vi "Add Stream.vi"(6 "Pixel Fornat || Options":u32, 8 "error in (no error)":errorcluster, 9 "Desired Stream Parameters":T1, 10 "Device ID":string, 11 "CameraManager":refnum<data-value>) -> (0 "error out":errorcluster, 2 "Stream":refnum<data-value>, 3 "CameraManager (duplicate)":refnum<data-value>)   [LabVIEW 2020, in "g_ar_toolkit.capture.lvlib" / "CameraManager.lvclass"]
uses:
  CameraManager.lvclass
  Stream Parameters.ctl
  CameraStream/CameraStream.lvclass
  CameraManager.lvclass/CameraManager.ctl
  bin/g_ar_toolkit.1.32.dll
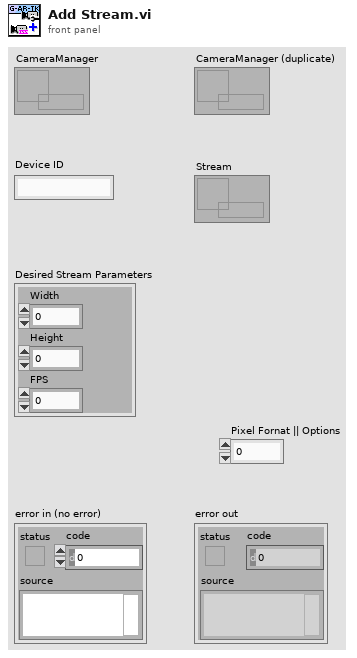
[diagram p1: front panel]
types:
  T1 = typedef "g_ar_toolkit.capture.lvlib/CameraManager.lvclass/Stream Parameters.ctl" = cluster{"Width":u16, "Height":u16, "FPS":u8}
  T2 = cluster{"Width":u32, "Height":u32, "FPS":u32, u32}
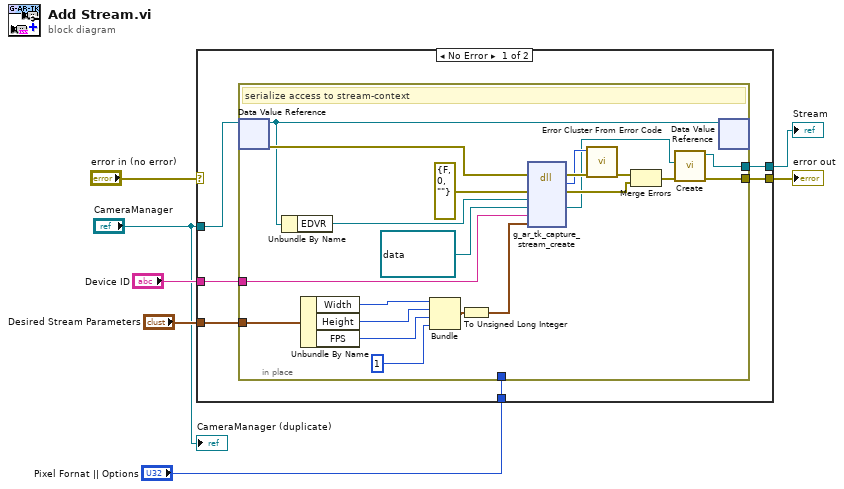
[diagram p0: block diagram]
diagram:
  n1 = case shown="No Error" "error in (no error)" {
    selector: "error in (no error)" -> [_ w35]
    tunnel: "CameraManager" -> [w13 _]
    tunnel: "Device ID" -> [w12 _]
    tunnel: "Desired Stream Parameters" -> [w11 _]
    tunnel: [w10 _] -> w4
    tunnel: [w9 w35] -> w3
    tunnel: "Pixel Fornat || Options" -> [w8 _]
    frame No Error {
      n2 = in-place {
        in-place-border: w12 -> [w30]
        in-place-border: w11 -> [w16]
        in-place-border: [w19] -> w10
        in-place-border: [w18] -> w9
        in-place-border: w8 -> [_]
        # "serialize access to stream-context"
        n3 = in-place-dvr #1(w13) -> (w17:refnum<class "CameraManager.lvclass">, w34:errorcluster)
        n4 = Unbundle By Name(w17) -> ("EDVR"=w32:refnum<data-value>)
        n5 = Unbundle By Name(w16) -> ("Width"=w28:u16, "Height"=w27:u16, "FPS"=w26:u8)
        n6 = Bundle("Width"=w28, "Height"=w27, "FPS"=w26, u8 1) -> (w29:cluster{"Width":u16, "Height":u16, "FPS":u8, u8})  [unwired: 1 in]
        n7 = To Unsigned Long Integer(number=w29) -> (unsigned 32bit integer=w15:T2)
        n8 = dll-call lib="C:/serenial/libraries/g-augmented-reality-toolkit/LabVIEW/bin/g_ar_toolkit.1.*.*" fn="g_ar_tk_capture_stream_create"(error in=w34, "error_cluster"=errorcluster {"status"=FALSE, "code"=0, "source"=""} ("error constant"), "EDVR_ctx"=w32, "EDVR_strm"=refnum<data-value> refnum ("EDVR"), "device_id"=w30, "stream_spec"=w15) -> (error out=w25:errorcluster, "MgErr"=w24:i32, "error_cluster"=w22:errorcluster, "EDVR_strm"=w20:refnum<data-value>)  [unwired: 5 in, 1 out]
        n9 = call <vilib>:"Error Cluster From Error Code.vi"("error in (no error)"=w25, "error code (0)"=w24) -> ("error out"=w23:errorcluster)  [unwired: 7 in]
        n10 = Merge Errors(w23, w22) -> (w21:errorcluster)
        n11 = call "Create.vi"("error in (no error)"=w21, "EDVR"=w20) -> ("error out"=w18:errorcluster, "Stream"=w19:refnum<data-value>)  [unwired: 8 in]
        n12 = in-place-dvr #1(w17) -> ()  [unwired: 2 out]
      }
    }
    frame Error {
    }
  }
  "error out" <- w3
  "Stream" <- w4
  "CameraManager (duplicate)" <- "CameraManager"
